vi "AddNextNode.vi"(6 "Variant in":variant, 7 "Shift Pressed?":bool, 8 "error in (no error)":errorcluster, 10 "QD Combo Box Ref":refnum<vi>, 11 "QD Launch VI Ref":refnum<vi>) -> (0 "error out":errorcluster, 4 "Variant out":variant)   [LabVIEW 2014]
doc: "Select a node and invoke this QD plugin to add the new node next to the selected node and connect the wires. It also clean the wires between these two nodes.\n\nDefault Shortcut - [N]"
panel:
  in  "Undo Name":string="Quick Drop Keyboard Shortcut"
  # "Do not change the connector pane of this VI.\n\nSee the block diagram for directions on how to use this template."
  # "Specify the name of the Undo transaction"
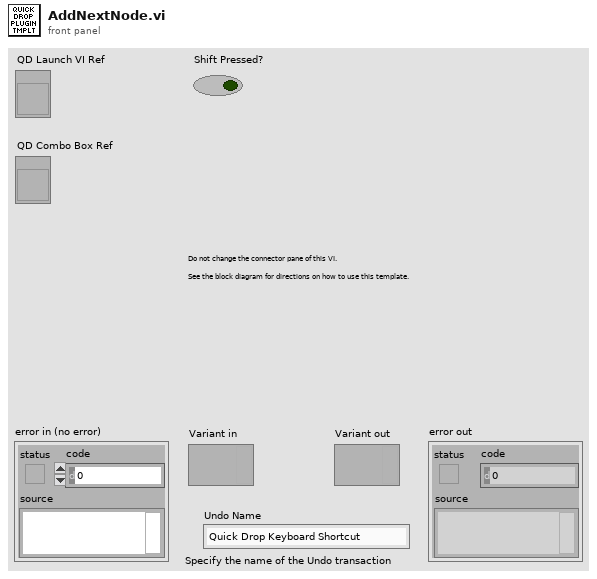
[diagram p1: front panel]
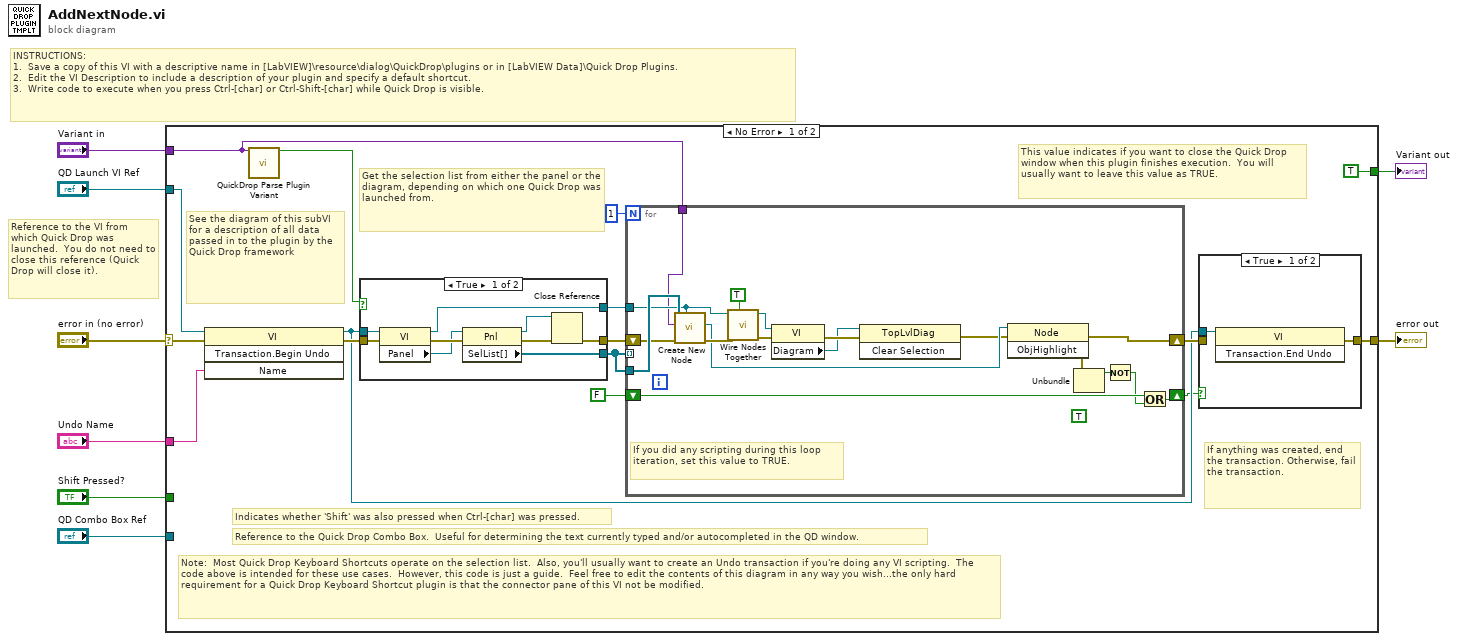
[diagram p0: block diagram]
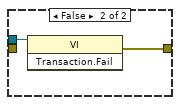
[diagram p2: hidden frame]
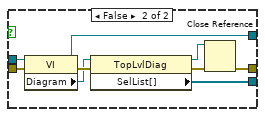
[diagram p3: hidden frame]
diagram:
  # "Reference to the VI from which Quick Drop was launched.  You do not need to close this reference (Quick Drop will close it)."
  # "INSTRUCTIONS:\n1.  Save a copy of this VI with a descriptive name in [LabVIEW]\\resource\\dialog\\QuickDrop\\plugins or in [LabVIEW Data]\\Quick Drop Plugins.\n2.  Edit the VI Description to include a description of your plugin and specify a default shortcut. \n3.  Write code to execute when you press Ctrl-[char] or Ctrl-Shift-[char] while Quick Drop is visible."
  n1 = case shown="No Error" "error in (no error)" {
    selector: "error in (no error)" -> [w24 w64]
    tunnel: [w18 w64] -> w7
    tunnel: "QD Launch VI Ref" -> [w23 _]
    tunnel: "Shift Pressed?" -> [_ _]
    tunnel: "QD Combo Box Ref" -> [_ _]
    tunnel: "Variant in" -> [w9 _]
    tunnel: "Undo Name" -> [w22 _]
    tunnel: [TRUE _] -> w1
    frame No Error {
      # "Note:  Most Quick Drop Keyboard Shortcuts operate on the selection list.  Also, you'll usually want to create an Undo transaction if you're doing any VI scripting.  The code above is intended for these use cases.  However, this code is just a guide.  Feel free to edit the contents of this diagram in any way you wish...the only hard requirement for a Quick Drop Keyboard Shortcut plugin is that the connector pane of this VI not be modified."
      # "Get the selection list from either the panel or the diagram, depending on which one Quick Drop was launched from."
      # "If anything was created, end the transaction. Otherwise, fail the transaction."
      # "This value indicates if you want to close the Quick Drop window when this plugin finishes execution.  You will usually want to leave this value as TRUE."
      # "See the diagram of this subVI for a description of all data passed in to the plugin by the Quick Drop framework"
      # "Reference to the Quick Drop Combo Box.  Useful for determining the text currently typed and/or autocompleted in the QD window."
      # "Indicates whether 'Shift' was also pressed when Ctrl-[char] was pressed."
      n2 = invoke class="VI" method="Transaction.Begin Undo"(reference=w23, error in=w24, "Name"=w22) -> (reference out=w15:refnum<vi>, error out=w19:errorcluster)  [unwired: 1 in, 2 out]
      n3 = call <vilib>:"QuickDrop Parse Plugin Variant.vi"("QDKS Variant in"=w9) -> ("QD Launch VI Panel?"=w20:bool)  [unwired: 12 in, 2 out]
      n4 = case shown="True" w20 {
        tunnel: w19 -> [w54 w63]
        tunnel: w15 -> [w53 w62]
        tunnel: [w48 w57] -> w17
        tunnel: [w47 w56] -> w11
        tunnel: [w46 w55] -> w10
        frame True {
          n5 = property class="VI"(reference=w53, error in=w54) -> (reference out=w46:refnum<vi>, error out=w52:errorcluster, "Panel"=w51:refnum<vi>)
          n6 = property class="Pnl"(reference=w51, error in=w52) -> (reference out=w49:refnum<vi>, error out=w50:errorcluster, "SelList[]"=w47:refnum<vi>[])
          n7 = Close Reference(reference=w49, error in (no error)=w50) -> (error out=w48:errorcluster)
        }
        frame False {
          n8 = property class="VI"(reference=w62, error in=w63) -> (reference out=w55:refnum<vi>, error out=w61:errorcluster, "Diagram"=w60:refnum<vi>)
          n9 = property class="TopLvlDiag"(reference=w60, error in=w61) -> (reference out=w58:refnum<vi>, error out=w59:errorcluster, "SelList[]"=w56:refnum<vi>[])
          n10 = Close Reference(reference=w58, error in (no error)=w59) -> (error out=w57:errorcluster)
        }
      }
      n11 = for {
        N: 1 -> [_]
        shift-right: [w33] -> w16
        shift-left: w17 -> [w36]
        shift-right: [w40] -> w13
        shift-left: FALSE -> [w41]
        tunnel: w11 -> [_] mode=indexing
        tunnel: w11 -> [w37]
        tunnel: w10 -> [w35]
        tunnel: w9 -> [w34]
        (unwired) TRUE ("x")
        # "If you did any scripting during this loop iteration, set this value to TRUE."
        n12 = call <resource>:"Create New Node.vi"("VI Ref"=w35, "error in (no error)"=w36, "Variant in"=w34, "SelList[]"=w37) -> ("error out"=w39:errorcluster, "Node Refnum"=w32:refnum<vi>)  [unwired: 5 in, 1 out]
        n13 = call <resource>:"Wire Nodes Together.vi"("Shift Pressed?"=TRUE, "error in (no error)"=w39, "VI Ref"=w35) -> ("error out"=w29:errorcluster, "dup VI"=w28:refnum<vi>)  [unwired: 7 in]
        n14 = property class="VI"(reference=w28, error in=w29) -> (error out=w27:errorcluster, "Diagram"=w25:refnum<vi>)  [unwired: 1 out]
        n15 = invoke class="TopLvlDiag" method="Clear Selection"(reference=w25, error in=w27) -> (error out=w26:errorcluster)  [unwired: 1 in, 2 out]
        n16 = invoke class="Node" method="ObjHighlight"(reference=w32, error in=w26) -> (error out=w33:errorcluster)  [unwired: 1 in, 2 out]
        n17 = Unbundle(w33) -> ("status"=w31:bool)  [unwired: 2 out]
        n18 = Not(x=w31) -> (.not. x?=w30:bool)
        n19 = Or(x=w41, y=w30) -> (x .or. y?=w40:bool)
      }
      n20 = case shown="True" w13 {
        tunnel: w15 -> [w42 w44]
        tunnel: [w43 w45] -> w18
        tunnel: w16 -> [_ _]
        frame True {
          n21 = invoke class="VI" method="Transaction.End Undo"(reference=w42) -> (error out=w43:errorcluster)  [unwired: 2 in, 2 out]
        }
        frame False {
          n22 = invoke class="VI" method="Transaction.Fail"(reference=w44) -> (error out=w45:errorcluster)  [unwired: 2 in, 2 out]
        }
      }
    }
    frame Error {
    }
  }
  "error out" <- w7
  "Variant out" <- w1
